vi "Get NotifyIcon Refernece.vi"(8 "error in (no error)":errorcluster) -> (0 "error out":errorcluster, 3 "reference out":T1)   [LabVIEW 2019, in "Test Bench Tools.lvlib"]
uses:
  Test Bench Tools.lvlib
  System.Windows.Forms
  System.Drawing
panel:
  in  "ico path":path=path "C:/Program Files (x86)/National Instruments/LabVIEW 2019/vi.lib/XXW Engineering/Test Bench Tools/Test Bench Manage.ico"
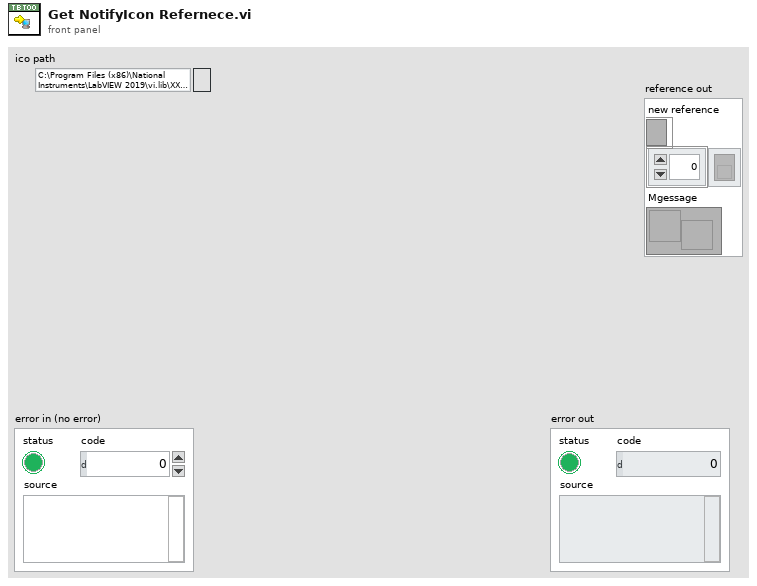
[diagram p1: front panel]
types:
  T1 = cluster{"new reference":refnum<k24>, "Array":refnum<k27>[], "Mgessage":refnum<user-event>}
  T2 = enum32{"invalid app kind", "Development System", "Run Time System", "Student Edition", "Embedded LabVIEW", "Evaluation", "Custom"}
  T3 = cluster{"new reference":refnum<k24>, refnum<k27>[], "Mgessage":refnum<user-event>}
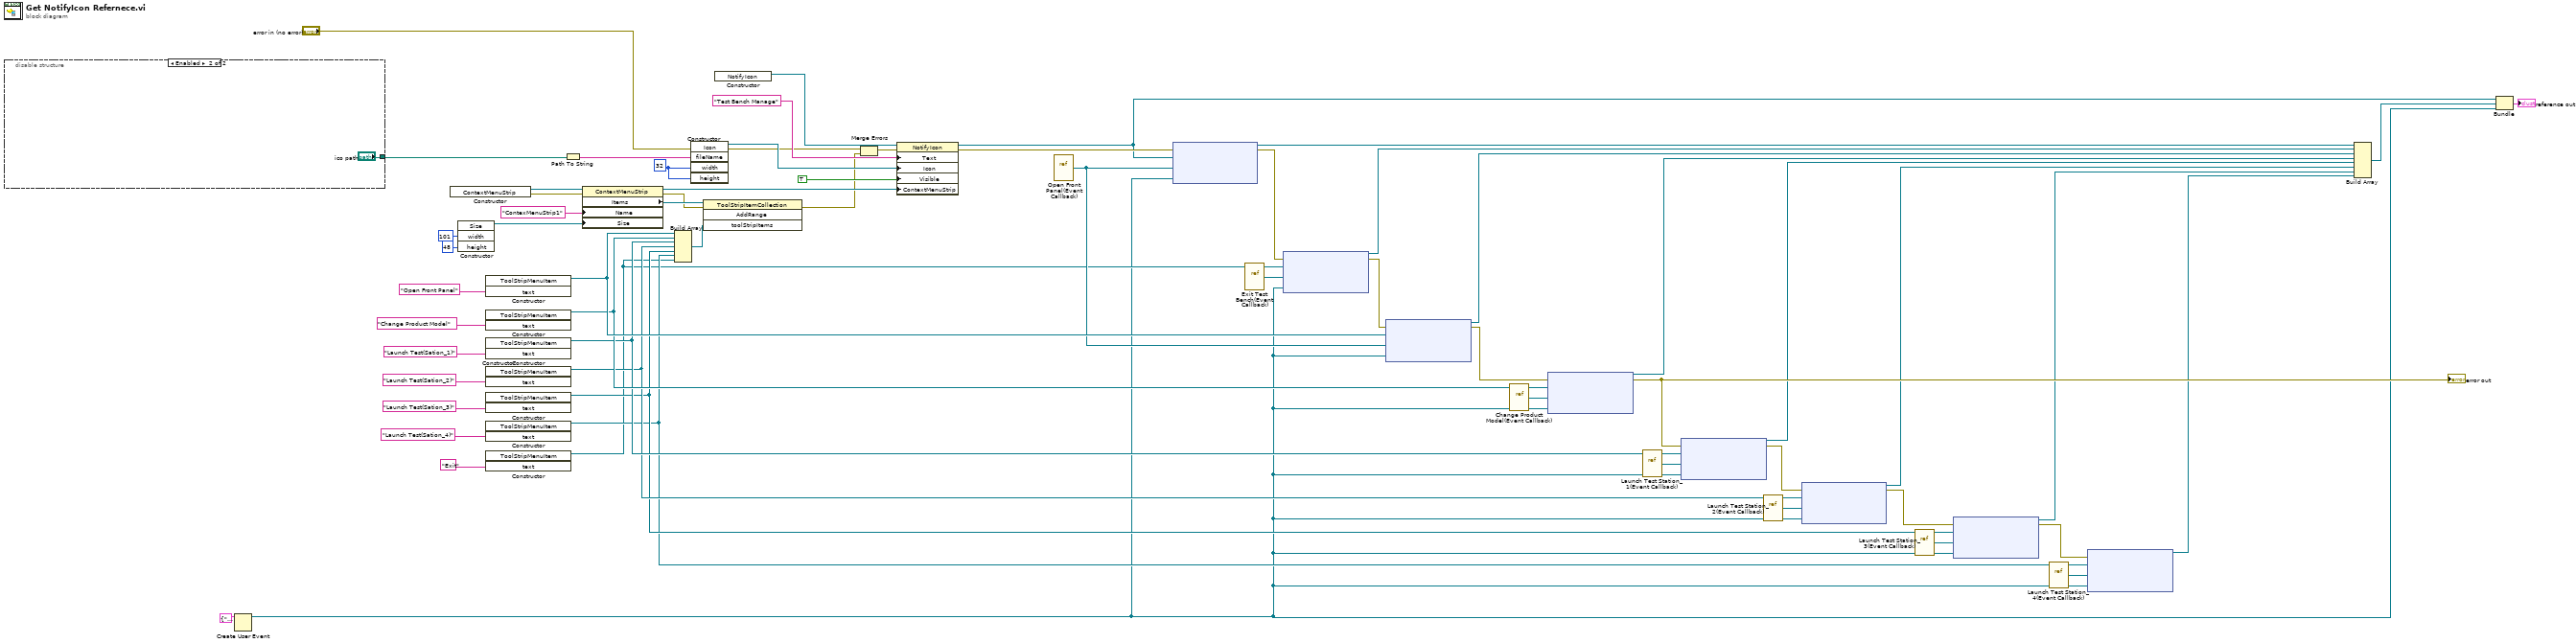
[diagram p0: block diagram]
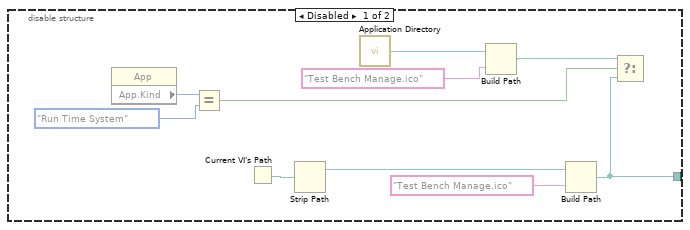
[diagram p2: hidden frame]
diagram:
  w63 = 32 ("width")
  n1 = disable-structure shown="Enabled" {
    disable-tunnel: [w70 "ico path"] -> w1
    frame Disabled {
      n2 = property class="App"() -> ("App.Kind"=w69:T2)  [unwired: 2 in, 2 out]
      n3 = Equal?(x=w69, y=T2."Run Time System" ("Application:Kind")) -> (x = y?=w67:bool)
      n4 = Current VI's Path() -> (path=w72:path)
      n5 = Strip Path(path=w72) -> (stripped path=w73:path)  [unwired: 1 out]
      n6 = call <vilib>:"Application Directory.vi"() -> ("Application Directory"=w66:path)
      n7 = Build Path(base path=w66, name or relative path="Test Bench Manage.ico") -> (appended path=w64:path)
      n8 = Build Path(base path=w73, name or relative path="Test Bench Manage.ico") -> (appended path=w70:path)
      n9 = Select(t=w64, s=w67, f=w70) -> ()  [unwired: 1 out]
    }
    frame Enabled {
    }
  }
  n10 = Create User Event(user event datatype=cluster{"Message":string, "Value":variant} {"Message"="", "Value"=variant} ("Mgessage")) -> (user event=w3:refnum<user-event>)  [unwired: 1 in, 1 out]
  n11 = constructor class="ContextMenuStrip"() -> (reference out=w55:refnum<k24>, error out=w47:errorcluster)  [unwired: 3 in, 1 out]
  n12 = constructor class="Size"("width"=101, "height"=48) -> (reference out=w51:refnum<k24>)  [unwired: 3 in, 4 out]
  n13 = constructor class="ToolStripMenuItem"("text"="Open Front Panel") -> (reference out=w39:refnum<k24>)  [unwired: 3 in, 3 out]
  n14 = constructor class="ToolStripMenuItem"("text"="Change Product Model") -> (reference out=w30:refnum<k24>)  [unwired: 3 in, 3 out]
  n15 = constructor class="ToolStripMenuItem"("text"="Launch Test(Sation_1)") -> (reference out=w20:refnum<k24>)  [unwired: 3 in, 3 out]
  n16 = constructor class="ToolStripMenuItem"("text"="Launch Test(Sation_2)") -> (reference out=w18:refnum<k24>)  [unwired: 3 in, 3 out]
  n17 = constructor class="ToolStripMenuItem"("text"="Launch Test(Sation_3)") -> (reference out=w16:refnum<k24>)  [unwired: 3 in, 3 out]
  n18 = constructor class="ToolStripMenuItem"("text"="Launch Test(Sation_4)") -> (reference out=w14:refnum<k24>)  [unwired: 3 in, 3 out]
  n19 = constructor class="ToolStripMenuItem"("text"="Exit") -> (reference out=w5:refnum<k24>)  [unwired: 3 in, 3 out]
  n20 = Path To String(path=w1) -> (string=w43:string)
  n21 = property class="ContextMenuStrip"(reference=w55, error in=w47, "Name"="ContexMenuStrip1", "Size"=w51) -> (reference out=w50:refnum<k24>, error out=w46:errorcluster, "Items"=w54:refnum<k24>)
  n22 = Build Array(w39, w30, w20, w18, w16, w14, w5) -> (w53:refnum<k24>[])
  n23 = constructor class="Icon"(error in="error in (no error)", "fileName"=w43, "width"=w63, "height"=w63) -> (reference out=w61:refnum<k24>, error out=w58:errorcluster)  [unwired: 2 in, 4 out]
  n24 = invoke class="ToolStripItemCollection" method="AddRange"(reference=w54, error in=w46, "toolStripItems"=w53) -> (error out=w44:errorcluster)  [unwired: 1 in, 3 out]
  n25 = constructor class="NotifyIcon"() -> (reference out=w59:refnum<k24>)  [unwired: 3 in, 2 out]
  n26 = Merge Errors(w58, w44) -> (w45:errorcluster)
  n27 = property class="NotifyIcon"(reference=w59, error in=w45, "Text"="Test Bench Manage", "Icon"=w61, "Visible"=TRUE, "ContextMenuStrip"=w50) -> (reference out=w27:refnum<k24>, error out=w41:errorcluster)
  n28 = vi-ref "Open Front Panel(Event Callback).vi"() -> ("vi reference"=w34:refnum<vi>)
  n29 = node(w41, w27, w34, w3) -> (w37:refnum<k27>, w40:errorcluster)  [unwired: 1 in]
  n30 = vi-ref "Exit Test Bench(Event Callback).vi"() -> ("vi reference"=w33:refnum<vi>)
  n31 = node(w40, w5, w33, w3) -> (w36:refnum<k27>, w38:errorcluster)  [unwired: 1 in]
  n32 = node(w38, w39, w34, w3) -> (w35:refnum<k27>, w31:errorcluster)  [unwired: 1 in]
  n33 = vi-ref "Change Product Model(Event Callback).vi"() -> ("vi reference"=w28:refnum<vi>)
  n34 = node(w31, w30, w28, w3) -> (w29:refnum<k27>, w21:errorcluster)  [unwired: 1 in]
  "error out" <- w21
  n35 = vi-ref "Launch Test Station_1(Event Callback).vi"() -> ("vi reference"=w9:refnum<vi>)
  n36 = node(w21, w20, w9, w3) -> (w13:refnum<k27>, w19:errorcluster)  [unwired: 1 in]
  n37 = vi-ref "Launch Test Station_2(Event Callback).vi"() -> ("vi reference"=w8:refnum<vi>)
  n38 = node(w19, w18, w8, w3) -> (w12:refnum<k27>, w17:errorcluster)  [unwired: 1 in]
  n39 = vi-ref "Launch Test Station_3(Event Callback).vi"() -> ("vi reference"=w7:refnum<vi>)
  n40 = node(w17, w16, w7, w3) -> (w11:refnum<k27>, w15:errorcluster)  [unwired: 1 in]
  n41 = vi-ref "Launch Test Station_4(Event Callback).vi"() -> ("vi reference"=w6:refnum<vi>)
  n42 = node(w15, w14, w6, w3) -> (w10:refnum<k27>)  [unwired: 1 in, 1 out]
  n43 = Build Array(w37, w36, w35, w29, w13, w12, w11, w10) -> (w26:refnum<k27>[])
  n44 = Bundle("new reference"=w27, w26, "Mgessage"=w3) -> (→"reference out":T3)  [unwired: 1 in]
